vi "About Box.vi"() -> ()   [LabVIEW 2015]
uses:
  Type/_RT Command.ctl
  Global.vi
panel:
  out "Software version":string="Ionica Firmware; FPGA: 277101103; RT: 341101125\n(System is idling: 0h3m24s)"
  out "version":string="Ionica Firmware; FPGA: 277101103; RT: 341101125\n(System is idling: 0h3m24s)"
  in  "OK":bool
  # "Copyright ©Aug. 12, 2016\nIonics Mass Spectrometry Group, Inc.\nAll Right Reserved\n\nAll Right Reserved"
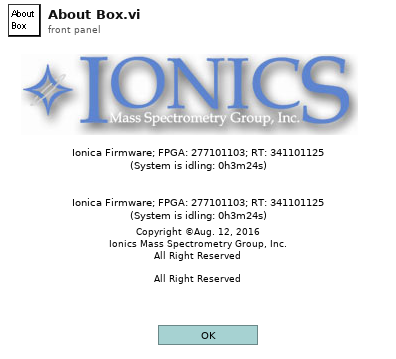
[diagram p1: front panel]
types:
  T1 = typedef "_RT Command.ctl" = enum16{"xml Start Run", "xml Start Actual Run", "xml Stop Run", "xml Runtime Update", "xml Get Status", "xml Get Table", "xml Set Table", "xml Get Configuration", "xml System Status", "xml Set LC Input Logic", "xml Get Data", "xml Get Info", "Start", "StartActualRun", "Stop", "Runtime Update", "Get Data", "Get Info", "Get Status", "Get Param", "Get Config", "Get Table", "Read ADC", "Set Oscillator", "Update Config", "Update Table", "Set All Pol", "Set Pol and DC", "Set Max Mass", "Toggle RP", "Toggle EL", "Set PIC", "Initialize Turbo", "Send Turbo Comm", "Close Turbo", "P1", "P2", "P3", "Send Serial", "Set LC Out", "Get LC In", "Read VAC", "Test Table", "Toggle Power", "Get Startup", "Set Startup", "Get ADC Table", "Set ADC Table", "Get Brief Status", "Get Detail Status", "Auxiliary Update", "Set CC Logics", "Set CC Input Logics", "Ignore Error", "invalid"}
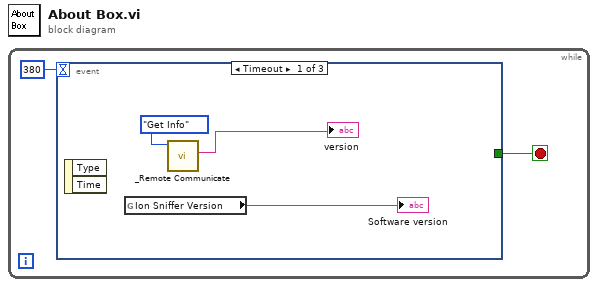
[diagram p0: block diagram]
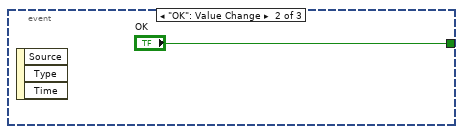
[diagram p2: hidden frame]
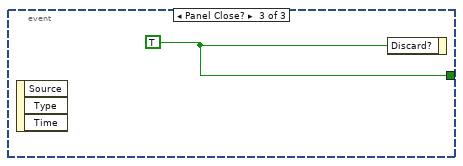
[diagram p3: hidden frame]
diagram:
  n1 = while {
    stop <- w1 stop-if-true
    n2 = event shown="[0] Timeout" {
      selector: _ -> [_ _ _]
      dyn-events: _ -> [_ _ _]
      timeout: 380 -> [_ _ _]
      tunnel: [_ "OK" w7] -> w1
      event Timeout {
        n3 = event-data() -> ()  [unwired: 3 out]
        n4 = global read "Global.vi" "Ion Sniffer Version"() -> (→"Software version":string)
        n5 = call "_Remote Communicate.vi"("Command"=_RT_Command."Get Info") -> ("Info"=→"version":string)  [unwired: 5 in, 3 out]
      }
      event "OK": Value Change {
        n6 = event-data() -> ()  [unwired: 4 out]
      }
      event Panel Close? {
        w7 = TRUE ("Discard?")
        n7 = event-data() -> ()  [unwired: 4 out]
        n8 = event-data("Discard?"=w7) -> ()  [unwired: 1 in, 1 out]
      }
    }
  }
